vi "Read firmware info.vi"(8 "error in (no error)":errorcluster, 11 "Refnum in":T1) -> (0 "error out":errorcluster, 2 "Fw Version":string, 3 "Refnum out":T1)   [LabVIEW 2015, in "7976R_v1.lvclass"]
uses:
  <userlib>/SE-APP-Receiver/NI5772/7976R_v1/7976R_v1.lvclass
  <userlib>/SE-APP-Receiver/NI5772/7976R_v1/Private/FPGA VI Reference_DDC_v1.8.ctl
  <vilib>/Utility/error.llb/Error Cluster From Error Code.vi
  <vilib>/rvi/errors/niLvFpgaAdjustHostInterfaceError.vi
  <vilib>/rvi/interface/nirviReadWriteControl/nirviReadWriteControl.xnode
  NiFpgaLv.dll
  <vilib>/rvi/interface/Simulation/niFpgaSimulationCallBeginRW.vi
panel:
  out "fw.err":bool
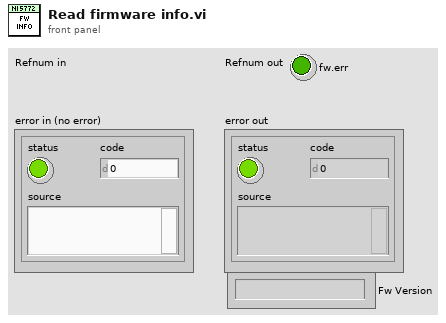
[diagram p1: front panel]
types:
  T1 = typedef "7976R_v1.lvclass/FPGA VI Reference_DDC_v1.8.ctl" = refnum<k20>
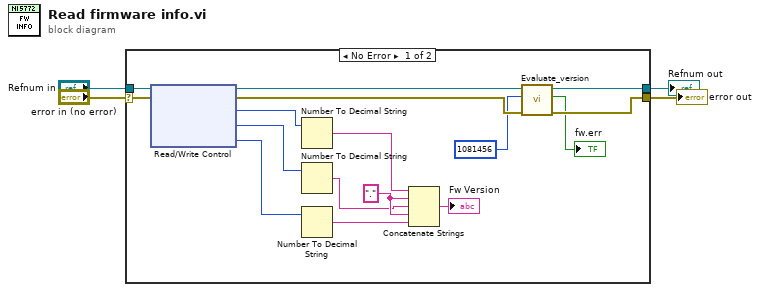
[diagram p0: block diagram]
diagram:
  n1 = case shown="No Error" "error in (no error)" {
    selector: "error in (no error)" -> [w19 w21]
    tunnel: "Refnum in" -> [w20 w22]
    tunnel: [w8 w22] -> w2
    tunnel: [w7 w21] -> w3
    frame No Error {
      w15 = "."
      n2 = xnode "Read/Write Control"("FPGA VI Reference In"=w20, "error in"=w19) -> ("FPGA VI Reference Out"=w10:T1, "error out"=w9:errorcluster, "ver.major"=w18:u8, "ver.technical"=w17:u8, "ver.editorial"=w16:u8)
      n3 = Number To Decimal String(number=w18) -> (decimal integer string=w14:string)  [unwired: 1 in]
      n4 = Number To Decimal String(number=w17) -> (decimal integer string=w13:string)  [unwired: 1 in]
      n5 = Number To Decimal String(number=w16) -> (decimal integer string=w12:string)  [unwired: 1 in]
      n6 = Concatenate Strings(w14, w15, w13, w15, w12) -> (→"Fw Version":string)
      n7 = call <userlib>:"Evaluate_version.vi"("error in (no error)"=w9, "min.expected"=u64 1081456, "Refnum in"=w10) -> ("error out"=w7:errorcluster, "dbg.lic.error"=→"fw.err":bool, "Refnum out"=w8:T1)  [unwired: 5 in, 1 out]
    }
    frame Error {
    }
  }
  "error out" <- w3
  "Refnum out" <- w2
